vi "Actor Core.vi"(8 "error in":errorcluster, 11 "CS++SimMotor in":refnum<class "CS++SimMotor.lvclass">) -> (0 "error out":errorcluster, 3 "Actor out":refnum<class "Actor.lvclass">)   [LabVIEW 2015, in "CS++SimMotor.lvlib" / "CS++SimMotor.lvclass"]
doc: "(<B>Filename</B>: Actor Framework.lvlib:Actor.lvclass:Actor Core.vi)\n\nReceives messages to the actor, reacts to them, and initiates any error handling that may shut the actor down.\n\nDescendant classes may override this VI to append parallel tasks for the actor to complete while it handles messages. Overrides use the Call Parent Method node."
uses:
  CS++SimMotor.lvclass
  <vilib>/ActorFramework/Actor/Actor.lvclass
  CSPP_Core/Actors/CS++BaseActor/CS++BaseActor.lvclass/CS++BaseActor.ctl
  CS++SimMotor.lvclass/CS++SimMotor.ctl
  CSPP_Core/Classes/CS++ProcessVariables/ProcessVariable/PV.lvclass
  CSPP_Core/Classes/CS++ProcessVariables/ProcessVariable/PV.lvclass/PV.ctl
  CSPP_Core/Classes/CS++ProcessVariables/ProcessVariable/Write Data.vi
  CSPP_Core/Classes/CS++ProcessVariables/ProcessVariable/Write Timestamp.vi
  CSPP_DeviceBase/CS++Motor/CS++Motor.lvclass
  CSPP_Core/Actors/CS++BaseActor/CS++BaseActor.lvclass
  CSPP_Core/Classes/CS++ProcessVariables/PVConnection/PVConnection.lvclass
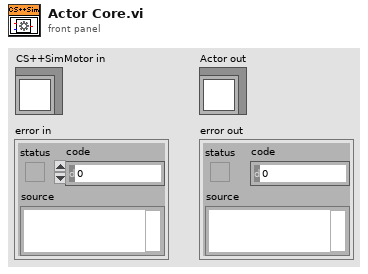
[diagram p1: front panel]
types:
  T1 = cluster{"RawSetPosition":dbl, "RawActPosition":dbl}
  T2 = cluster{"Stop Event":refnum<user-event>, "Pos Update Event":refnum<user-event>, "Reset Event":refnum<user-event>}
  T3 = cluster{"RawSetPosition":dbl, "RawActPosition":dbl}[]
  T4 = enum16{"RelativeMovement", "AbsoluteMovement", "Stop", "ReferenceMovement"}
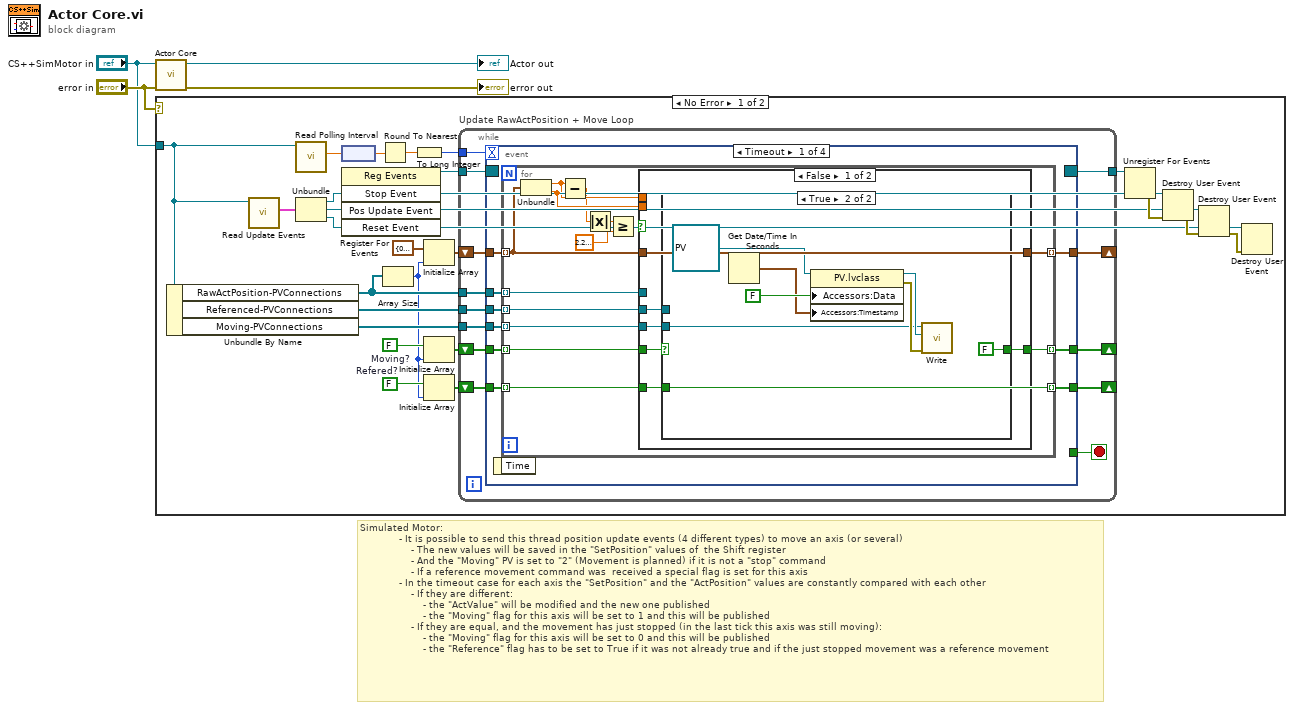
[diagram p0: block diagram]
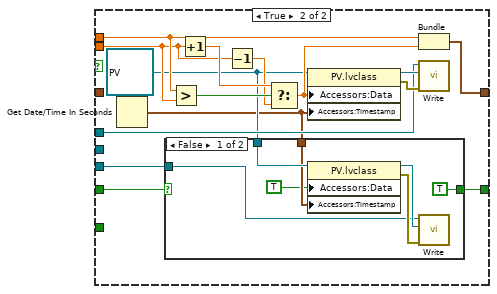
[diagram p3: hidden frame]
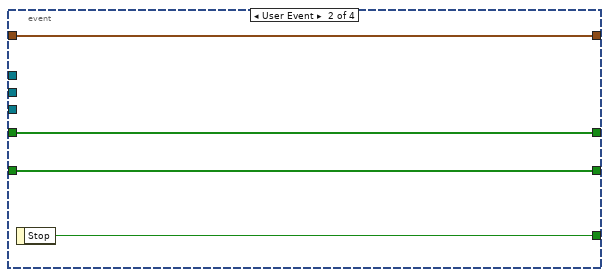
[diagram p5: hidden frame]
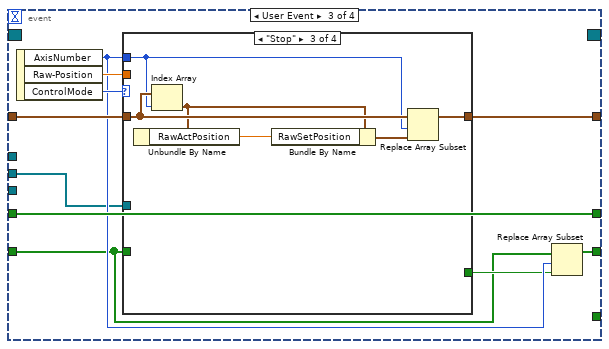
[diagram p6: hidden frame]
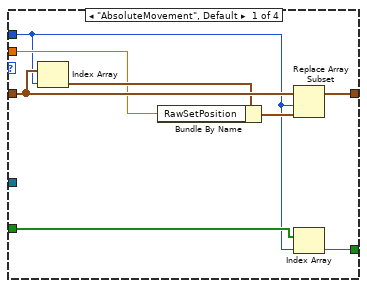
[diagram p7: hidden frame]
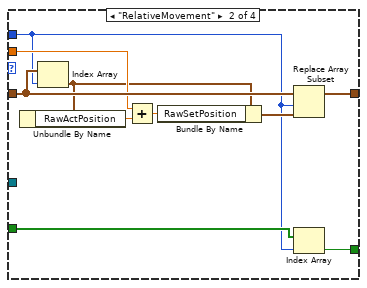
[diagram p8: hidden frame]
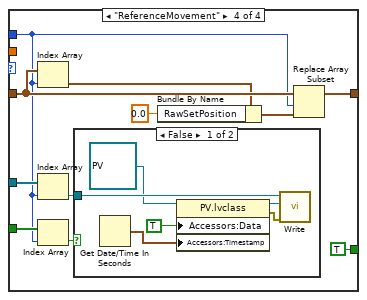
[diagram p9: hidden frame]
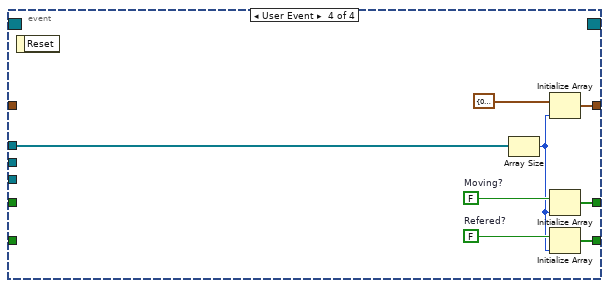
[diagram p11: hidden frame]
diagram:
  # "Simulated Motor: \n             - It is possible to send this thread position update events (4 different types) to move an axis (or several)\n                 - The new values will be saved in the \"SetPosition\" values of  the Shift register\n                 - And the \"Moving\" PV is set to \"2\" (Movement is planned) if it is not a \"stop\" command\n                 - If a reference movement command was  received a special flag is set for this axis\n             - In the timeout case for each axis the \"SetPosition\" and the \"ActPosition\" values are constantly compared with each other\n                 - If they are different: \n                     - the \"ActValue\" will be modified and the new one published \n                     - the \"Moving\" flag for this axis will be set to 1 and this will be published\n                 - If they are equal, and the movement has just stopped (in the last tick this axis was still moving):\n                     - the \"Moving\" flag for this axis will be set to 0 and this will be published\n                     - the \"Reference\" flag has to be set to True if it was not already true and if the just stopped movement was a reference movement"
  n1 = call-parent "Actor Core.vi"("error in"="error in", "CS++Motor in"="CS++SimMotor in") -> ("error out"=→"error out":errorcluster, "Actor out"=→"Actor out":refnum<class "Actor.lvclass">)  [unwired: 8 in]
  n2 = case shown="No Error" "error in" {
    tunnel: "CS++SimMotor in" -> [w22 _]
    frame No Error {
      w9 = FALSE  # Refered?
      w12 = FALSE  # Moving?
      n3 = Unbundle By Name(w22) -> ("RawActPosition-PVConnections"=w10:refnum<class "PVConnection.lvclass">[], "Referenced-PVConnections"=w14:refnum<class "PVConnection.lvclass">[], "Moving-PVConnections"=w11:refnum<class "PVConnection.lvclass">[])
      n4 = call "Read Update Events.vi"("CS++SimMotor in"=w22) -> ("Update Events"=w23:T2)  [unwired: 8 in, 2 out]
      n5 = call "Read Polling Interval.vi"("CS++BaseActor in"=w22) -> ("Polling Interval"=w26:dbl[unit])  [unwired: 8 in, 2 out]
      n6 = Unbundle(w23) -> ("Stop Event"=w18:refnum<user-event>, "Pos Update Event"=w17:refnum<user-event>, "Reset Event"=w5:refnum<user-event>)
      n7 = node(w26) -> (w27:dbl)
      n8 = register-events(w18, w17, w5) -> (reference out=w24:refnum<event-registration>)  [unwired: 2 in, 1 out]
      n9 = Round To Nearest(number=w27) -> (nearest integer value=w28:dbl)
      n10 = Array Size(array=w10) -> (size(s)=w7:i32)
      n11 = To Long Integer(number=w28) -> (32bit integer=w25:i32)
      n12 = Initialize Array(T1 {"RawSetPosition"=0.0, "RawActPosition"=0.0}, w7) -> (w16:T3)
      n13 = Initialize Array(w12, w7) -> (w13:bool[])
      n14 = Initialize Array(w9, w7) -> (w8:bool[])
      n15 = while "Update RawActPosition + Move Loop" {
        tunnel: w25 -> [w41]
        tunnel: w24 -> [w40]
        shift-right: [w37] -> _
        shift-left: w16 -> [w38]
        tunnel: w10 -> [w36]
        tunnel: [w35] -> w19
        tunnel: w14 -> [w34]
        shift-right: [w32] -> _
        shift-left: w13 -> [w33]
        tunnel: w11 -> [w31]
        shift-right: [w29] -> _
        shift-left: w8 -> [w30]
        stop <- w39 stop-if-true
        n16 = event shown="[0] Timeout" {
          selector: w40 -> [_ _ _ _]
          dyn-events: [_ _ _ _] -> w35
          timeout: w41 -> [_ _ _ _]
          tunnel: [_ w105 _ _] -> w39
          tunnel: w38 -> [w50 w104 w114 _]
          tunnel: [w49 w104 w115 w164] -> w37
          tunnel: w36 -> [w48 _ _ w158]
          tunnel: w34 -> [w47 _ w107 _]
          tunnel: w33 -> [w46 w103 w112 _]
          tunnel: [w45 w103 w112 w163] -> w32
          tunnel: w31 -> [w44 _ _ _]
          tunnel: w30 -> [w43 w102 w106 _]
          tunnel: [w42 w102 w110 w162] -> w29
          event Timeout {
            n17 = event-data() -> ()  [unwired: 1 in, 1 out]
            n18 = for {
              tunnel: w50 -> [w64] mode=indexing
              tunnel: [w63] -> w49 mode=indexing
              tunnel: w48 -> [w62] mode=indexing
              tunnel: w47 -> [w61] mode=indexing
              tunnel: w46 -> [w60] mode=indexing
              tunnel: [w59] -> w45 mode=indexing
              tunnel: w44 -> [w58] mode=indexing
              tunnel: w43 -> [w57] mode=indexing
              tunnel: [w57] -> w42 mode=indexing
              n19 = Unbundle(w64) -> ("RawSetPosition"=w56:dbl, "RawActPosition"=w55:dbl)
              n20 = Subtract(x=w56, y=w55) -> (x-y=w54:dbl)
              n21 = Absolute Value(x=w54) -> (abs(x)=w53:dbl)
              n22 = Greater Or Equal?(x=w53, y=2.220446049250313e-16) -> (x >= y?=w52:bool)
              n23 = case shown="False" w52 {
                tunnel: w55 -> [_ w85]
                tunnel: w56 -> [_ w87]
                tunnel: w64 -> [w70 _]
                tunnel: [w70 w91] -> w63
                tunnel: w62 -> [_ w90]
                tunnel: w61 -> [w66 _]
                tunnel: w60 -> [w69 w81]
                tunnel: [w68 w80] -> w59
                tunnel: w58 -> [w67 w79]
                tunnel: w57 -> [w65 _]
                frame False {
                  n24 = case shown="True" w69 {
                    selector: w69 -> [w71 _]
                    tunnel: [w71 FALSE] -> w68
                    tunnel: w67 -> [_ w76]
                    tunnel: w66 -> [_ _]
                    tunnel: w65 -> [_ _]
                    frame False {
                    }
                    frame True {
                      n25 = Get Date/Time In Seconds() -> (seconds since 1Jan1904=w72:timestamp)
                      n26 = property class="PV.lvclass"(reference=refnum<class "PV.lvclass"> refnum ("PV"), "Accessors:Data"=FALSE, "Accessors:Timestamp"=w72) -> (reference out=w77:refnum<class "PV.lvclass">, error out=w78:errorcluster)  [unwired: 1 in]
                      n27 = call "Write.vi"("error in (no error)"=w78, "PV"=w77, "PVConnection in"=w76) -> ()  [unwired: 7 in, 2 out]
                    }
                  }
                }
                frame True {
                  w83 = refnum<class "PV.lvclass"> refnum ("PV")
                  n28 = Get Date/Time In Seconds() -> (seconds since 1Jan1904=w82:timestamp)
                  n29 = case shown="False" w81 {
                    selector: w81 -> [_ w101]
                    tunnel: w83 -> [w98 _]
                    tunnel: w82 -> [w97 _]
                    tunnel: [TRUE w101] -> w80
                    tunnel: w79 -> [w95 _]
                    frame False {
                      n30 = property class="PV.lvclass"(reference=w98, "Accessors:Data"=TRUE, "Accessors:Timestamp"=w97) -> (reference out=w99:refnum<class "PV.lvclass">, error out=w100:errorcluster)  [unwired: 1 in]
                      n31 = call "Write.vi"("error in (no error)"=w100, "PV"=w99, "PVConnection in"=w95) -> ()  [unwired: 7 in, 2 out]
                    }
                    frame True {
                    }
                  }
                  n32 = Greater?(x=w87, y=w85) -> (0:w88:bool)
                  n33 = Increment(x=w85) -> (x+1=w86:dbl)
                  n34 = Decrement(x=w85) -> (x-1=w84:dbl)
                  n35 = Select(t=w86, s=w88, f=w84) -> (s? t:f=w89:dbl)
                  n36 = property class="PV.lvclass"(reference=w83, "Accessors:Data"=w89, "Accessors:Timestamp"=w82) -> (reference out=w92:refnum<class "PV.lvclass">, error out=w93:errorcluster)  [unwired: 1 in]
                  n37 = Bundle("RawSetPosition"=w87, w89) -> (w91:cluster{"RawSetPosition":dbl, dbl})  [unwired: 1 in]
                  n38 = call "Write.vi"("error in (no error)"=w93, "PV"=w92, "PVConnection in"=w90) -> ()  [unwired: 7 in, 2 out]
                }
              }
            }
          }
          event User Event {
            n39 = event-data() -> ("Stop"=w105:bool)  [unwired: 1 in]
          }
          event User Event {
            n40 = event-data() -> ("AxisNumber"=w109:u8, "Raw-Position"=w113:dbl, "ControlMode"=w111:T4)  [unwired: 1 in]
            n41 = case shown="\"Stop\"" w111 {
              tunnel: [w123 w133 w139 w150] -> w115
              tunnel: w114 -> [w122 w132 w138 w149]
              tunnel: w109 -> [w117 w124 w137 w141]
              tunnel: w113 -> [w119 w129 _ _]
              tunnel: [w116 w125 _ TRUE ("ActRef?")] -> w108
              tunnel: w107 -> [_ _ _ w144]
              tunnel: w106 -> [w118 w126 _ w142]
              frame "AbsoluteMovement", Default {
                n42 = Index Array(array=w122, index=w117) -> (element=w121:T1)
                n43 = Bundle By Name(cluster=w121, "RawSetPosition"=w119) -> (w120:T1)
                n44 = Replace Array Subset(array=w122, new element=w120, index=w117) -> (w123:T3)
                n45 = Index Array(array=w118, index=w117) -> (element=w116:bool)
              }
              frame "RelativeMovement" {
                n46 = Index Array(array=w132, index=w124) -> (element=w128:T1)
                n47 = Unbundle By Name(w128) -> ("RawActPosition"=w127:dbl)
                n48 = Add(x=w129, y=w127) -> (x+y=w130:dbl)
                n49 = Bundle By Name(cluster=w128, "RawSetPosition"=w130) -> (w131:T1)
                n50 = Replace Array Subset(array=w132, new element=w131, index=w124) -> (w133:T3)
                n51 = Index Array(array=w126, index=w124) -> (element=w125:bool)
              }
              frame "Stop" {
                n52 = Index Array(array=w138, index=w137) -> (element=w135:T1)
                n53 = Unbundle By Name(w135) -> ("RawActPosition"=w134:dbl)
                n54 = Bundle By Name(cluster=w135, "RawSetPosition"=w134) -> (w136:T1)
                n55 = Replace Array Subset(array=w138, new element=w136, index=w137) -> (w139:T3)
              }
              frame "ReferenceMovement" {
                n56 = Index Array(array=w149, index=w141) -> (element=w147:T1)
                n57 = Index Array(array=w144, index=w141) -> (element=w143:refnum<class "PVConnection.lvclass">)
                n58 = Index Array(array=w142, index=w141) -> (element=w140:bool)
                n59 = case shown="False" w140 {
                  tunnel: w143 -> [w154 _]
                  frame False {
                    n60 = Get Date/Time In Seconds() -> (seconds since 1Jan1904=w152:timestamp)
                    n61 = property class="PV.lvclass"(reference=refnum<class "PV.lvclass"> refnum ("PV"), "Accessors:Data"=TRUE, "Accessors:Timestamp"=w152) -> (reference out=w156:refnum<class "PV.lvclass">, error out=w155:errorcluster)  [unwired: 1 in]
                    n62 = call "Write.vi"("error in (no error)"=w155, "PV"=w156, "PVConnection in"=w154) -> ()  [unwired: 7 in, 2 out]
                  }
                  frame True {
                  }
                }
                n63 = Bundle By Name(cluster=w147, "RawSetPosition"=0.0) -> (w148:T1)
                n64 = Replace Array Subset(array=w149, new element=w148, index=w141) -> (w150:T3)
              }
            }
            n65 = Replace Array Subset(array=w106, new element=w108, index=w109) -> (w110:bool[])
          }
          event User Event {
            w161 = FALSE  # Refered?
            w160 = FALSE  # Moving?
            n66 = event-data() -> ()  [unwired: 1 in, 1 out]
            n67 = Array Size(array=w158) -> (size(s)=w157:i32)
            n68 = Initialize Array(T1 {"RawSetPosition"=0.0, "RawActPosition"=0.0}, w157) -> (w164:T3)
            n69 = Initialize Array(w160, w157) -> (w163:bool[])
            n70 = Initialize Array(w161, w157) -> (w162:bool[])
          }
        }
      }
      n71 = Unregister For Events(event registration refnum=w19) -> (error out=w21:errorcluster)  [unwired: 1 in]
      n72 = Destroy User Event(user event=w18, error in=w21) -> (error out=w20:errorcluster)
      n73 = Destroy User Event(user event=w17, error in=w20) -> (error out=w6:errorcluster)
      n74 = Destroy User Event(user event=w5, error in=w6) -> ()  [unwired: 1 out]
    }
    frame Error {
    }
  }
